vi "ACC Login Dialog.vi"(5 "False Text (Cancel)":string="Cancel", 11 "Error in (no error)":errorcluster) -> (10 "Cancelled":bool, 15 "Error Out":errorcluster)   [LabVIEW 2011]
uses:
  Type Defs/ACTL Configuration Operation Enum.ctl
  Type Defs/ACTL Access Level Enum.ctl
panel:
  in  "Username":string(combo)
  in  "Cancel":bool
  in  "Login":bool
  in  "Password":string
  # "Login"
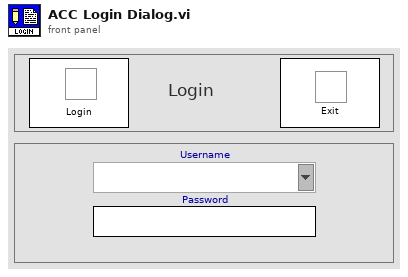
[diagram p1: front panel]
types:
  T1 = typedef "ACTL Configuration Operation Enum.ctl" = enum16{"Initialize", "Get Status", "Read", "Write", "Update", "Copy", "Edit"}
  T2 = typedef "ACTL Access Level Cluster.ctl" = cluster{"Operator":T3}
  T3 = typedef "ACTL Operator Cluster.ctl" = cluster{"Full Name":string, "Access Level":T4, "Name Set":string[], "Login":bool, "Password Set":string[]}
  T4 = typedef "ACTL Access Level Enum.ctl" = enum16{"Operator", "Technician", "Engineer", "Programmer"}
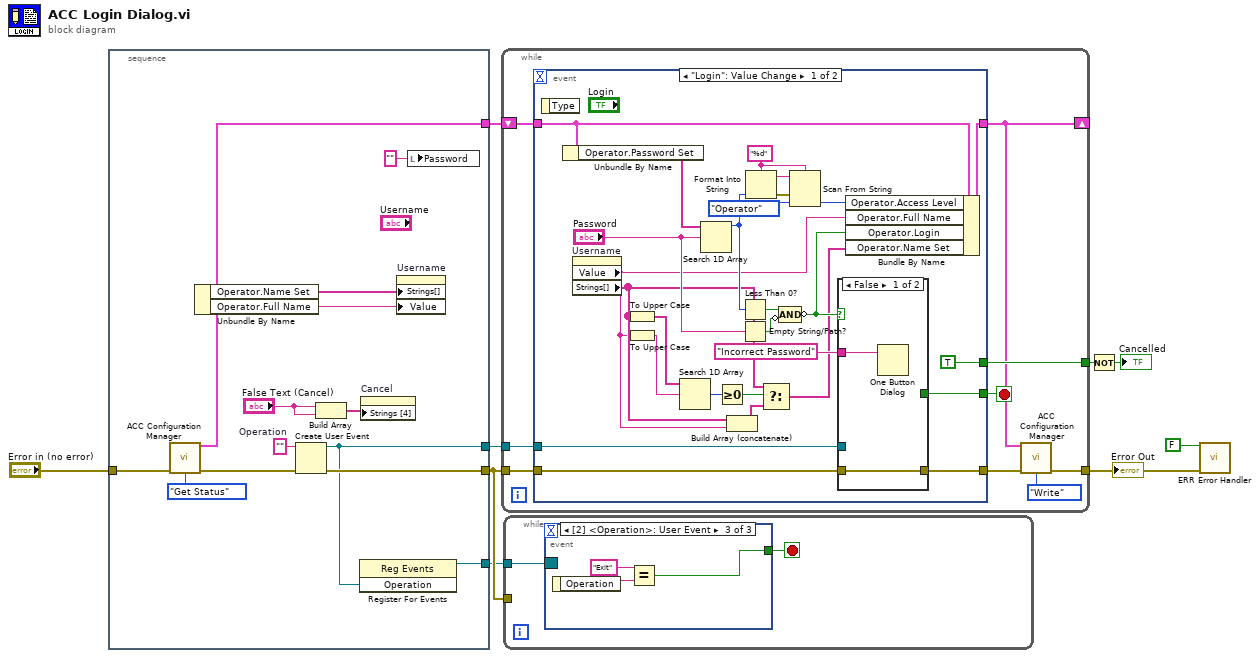
[diagram p0: block diagram]
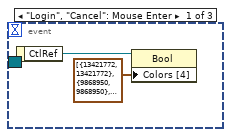
[diagram p2: hidden frame]
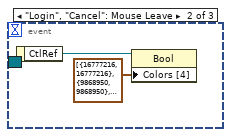
[diagram p3: hidden frame]
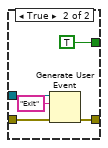
[diagram p4: hidden frame]
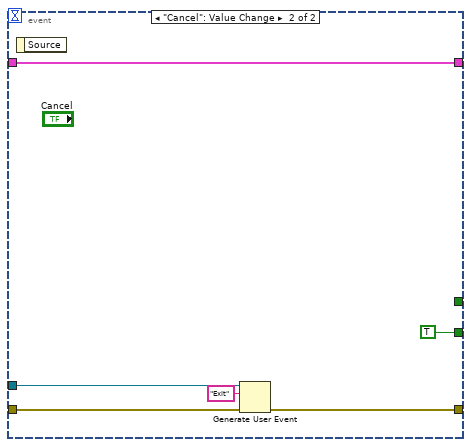
[diagram p5: hidden frame]
diagram:
  n1 = stacked-sequence {
    tunnel: [w10] -> w6
    tunnel: [w19] -> w4
    tunnel: "Error in (no error)" -> [w13]
    tunnel: [w17] -> w2
    tunnel: [w16] -> w1
    frame #0 {
      w18 = ""  # Operation
      n2 = call "ACC Configuration Manager.vi"("Error In (no error)"=w13, "Operation"=ACTL_Configuration_Operation_Enum."Get Status") -> ("System Configuration Out"=w10:T2, "Error Out"=w12:errorcluster)  [unwired: 3 in, 9 out]
      n3 = Unbundle By Name(w10) -> ("Operator.Name Set"=w15:string[], "Operator.Full Name"=w14:string)
      n4 = Create User Event(user event datatype=w18, error in=w12) -> (user event=w17:refnum<user-event>, error out=w19:errorcluster)
      n5 = Build Array("False Text (Cancel)", "False Text (Cancel)") -> (w20:string[])
      n6 = register-events(w17) -> (reference out=w16:refnum<event-registration>)  [unwired: 2 in, 1 out]
      n7 = property on="Cancel" class="Bool"("Strings [4]"=w20) -> ()  [unwired: 2 in, 2 out]
      n8 = property on="Username" class="CmbBox"("Strings[]"=w15, "Value"=w14) -> ()  [unwired: 2 in, 2 out]
      n9 = local write "Password"("" ("Password")) -> ()
    }
  }
  n10 = while {
    tunnel: [w25] -> w8
    tunnel: w4 -> [w30]
    shift-left: w6 -> [w31]
    shift-right: [w23] -> _
    tunnel: [w28] -> w9
    tunnel: w2 -> [w27]
    stop <- w29 stop-if-true
    n11 = event shown="[0] \"Login\": Value Change" {
      selector: _ -> [_ _]
      dyn-events: _ -> [_ _]
      timeout: _ -> [_ _]
      tunnel: w31 -> [w47 w66]
      tunnel: [w46 w66] -> w23
      tunnel: w30 -> [w43 w69]
      tunnel: [w42 w68] -> w26
      tunnel: [w45 TRUE] -> w29
      tunnel: [TRUE _] -> w28
      tunnel: w27 -> [w41 w67]
      event "Login": Value Change {
        w58 = "%d" ("Format String")
        n12 = event-data() -> ()  [unwired: 2 out]
        n13 = Unbundle By Name(w47) -> ("Operator.Password Set"=w49:string[])
        n14 = property on="Username" class="CmbBox"() -> ("Value"=w33:string, "Strings[]"=w34:string[])  [unwired: 2 in, 2 out]
        n15 = To Upper Case(1:w34) -> (0:w39:string[])
        n16 = To Upper Case(1:w33) -> (0:w38:string)
        n17 = Search 1D Array(1D array=w39, element=w38) -> (index of element=w37:i32)  [unwired: 1 out]
        n18 = Search 1D Array(1D array=w49, element="Password") -> (index of element=w53:i32)  [unwired: 1 out]
        n19 = Greater Or Equal To 0?(x=w37) -> (x >= 0?=w36:bool)
        n20 = Build Array (concatenate)(w34, w33) -> (w32:string[])
        n21 = Less Than 0?(x=w53) -> (x < 0?=w50:bool)
        n22 = Empty String/Path?(string/path="Password") -> (empty?=w51:bool)
        n23 = Format Into String(format string=w58, w53) -> (resulting string=w55:string, error out=w54:errorcluster)  [unwired: 2 in]
        n24 = Select(t=w34, s=w36, f=w32) -> (s? t:f=w35:string[])
        n25 = Compound Arithmetic op=AND(w50, invert w51) -> (invert w52:bool)
        n26 = Scan From String(format string=w58, input string=w55, error in=w54, default 1=ACTL_Access_Level_Enum."Operator" ("Access Level")) -> (output 1=w57:T4)  [unwired: 1 in, 3 out]
        n27 = case shown="False" w52 {
          tunnel: "Incorrect Password" ("message") -> [w59 _]
          tunnel: [_ TRUE] -> w45
          tunnel: w43 -> [w60 w64]
          tunnel: [w60 w63] -> w42
          tunnel: w41 -> [_ w62]
          frame False {
            n28 = One Button Dialog(message=w59) -> ()  [unwired: 2 out]
          }
          frame True {
            n29 = Generate User Event(user event=w62, event data cluster="Exit" ("event data"), error in=w64) -> (error out=w63:errorcluster)  [unwired: 1 out]
          }
        }
        n30 = Bundle By Name(cluster=w47, "Operator.Access Level"=w57, "Operator.Full Name"=w33, "Operator.Login"=w52, "Operator.Name Set"=w35) -> (w46:T2)
      }
      event "Cancel": Value Change {
        n31 = event-data() -> ()  [unwired: 2 out]
        n32 = Generate User Event(user event=w67, event data cluster="Exit" ("event data"), error in=w69) -> (error out=w68:errorcluster)  [unwired: 1 out]
      }
    }
    n33 = call "ACC Configuration Manager.vi"("System Configuration In (Write, Update Only)"=w23, "Error In (no error)"=w26, "Operation"=ACTL_Configuration_Operation_Enum."Write") -> ("Error Out"=w25:errorcluster)  [unwired: 2 in, 10 out]
  }
  "Error Out" <- w8
  n34 = while {
    tunnel: w4 -> [_]
    tunnel: w1 -> [w72]
    stop <- w73 stop-if-true
    n35 = event shown="[2] <Operation>: User Event" {
      selector: w72 -> [_ _ _]
      dyn-events: _ -> [_ _ _]
      timeout: _ -> [_ _ _]
      tunnel: [_ _ w78] -> w73
      event "Login", "Cancel": Mouse Enter {
        n36 = event-data() -> ("CtlRef"=w74:refnum<vi>)  [unwired: 1 out]
        n37 = property class="Bool"(reference=w74, "Colors [4]"=cluster{u32, u32}[] [{13421772, 13421772}, {9868950, 9868950}, {6710886, 6710886}, {9868950, 9868950}]) -> ()  [unwired: 1 in, 2 out]
      }
      event "Login", "Cancel": Mouse Leave {
        n38 = event-data() -> ("CtlRef"=w76:refnum<vi>)  [unwired: 1 out]
        n39 = property class="Bool"(reference=w76, "Colors [4]"=cluster{u32, u32}[] [{16777216, 16777216}, {9868950, 9868950}, {6710886, 6710886}, {9868950, 9868950}]) -> ()  [unwired: 1 in, 2 out]
      }
      event User Event {
        n40 = event-data() -> ("Operation"=w80:string)  [unwired: 1 out]
        n41 = Equal?(x="Exit", y=w80) -> (x = y?=w78:bool)
      }
    }
  }
  n42 = Not(x=w9) -> (.not. x?=→"Cancelled":bool)
  n43 = call "ERR Error Handler.vi"("Error Status"=FALSE ("Error Flag"), "Error In (no error)"=w8) -> ()  [unwired: 4 in, 10 out]
